vi "read_access_codes_from_file.vi"(8 "error in (no error)":errorcluster, 11 "Paths":cluster{"Access":path, "Refresh":path}) -> (0 "error out":errorcluster, 3 "Codes":cluster{"Access":string, "Refresh":string})   [LabVIEW 2016]
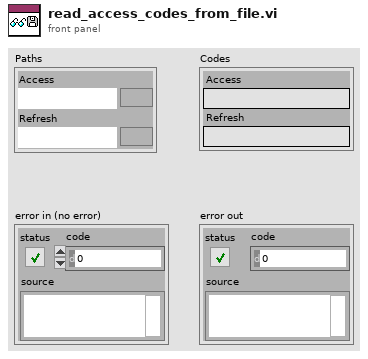
[diagram p1: front panel]
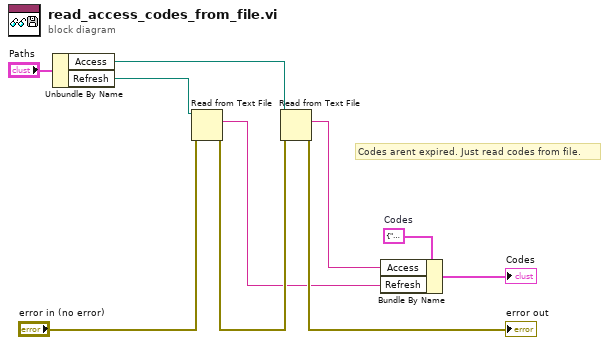
[diagram p0: block diagram]
diagram:
  w10 = cluster{"Access":string, "Refresh":string} {"Access"="", "Refresh"=""}  # Codes
  # "Codes arent expired. Just read codes from file."
  n1 = Unbundle By Name("Paths") -> ("Access"=w5:path, "Refresh"=w2:path)
  n2 = Read from Text File(file (use dialog)=w2, error in="error in (no error)") -> (text=w1:string, error out=w3:errorcluster)  [unwired: 2 in, 2 out]
  n3 = Read from Text File(file (use dialog)=w5, error in=w3) -> (text=w8:string, error out=→"error out":errorcluster)  [unwired: 2 in, 2 out]
  n4 = Bundle By Name(cluster=w10, "Access"=w8, "Refresh"=w1) -> (→"Codes":cluster{"Access":string, "Refresh":string})
